vi "Get_Coordinate System.vi"(8 "error in (no error)":errorcluster, 11 "SoftmotionAxis in":refnum<class "SoftmotionAxis.lvclass">) -> (0 "error out":errorcluster, 2 "Coordinate System":refnum<k21>, 3 "SoftmotionAxis out":refnum<class "SoftmotionAxis.lvclass">)   [LabVIEW 2017, in "SoftmotionAxis.lvclass"]
uses:
  SoftmotionAxis.lvclass
  SoftmotionAxis.lvclass/SoftmotionAxis.ctl
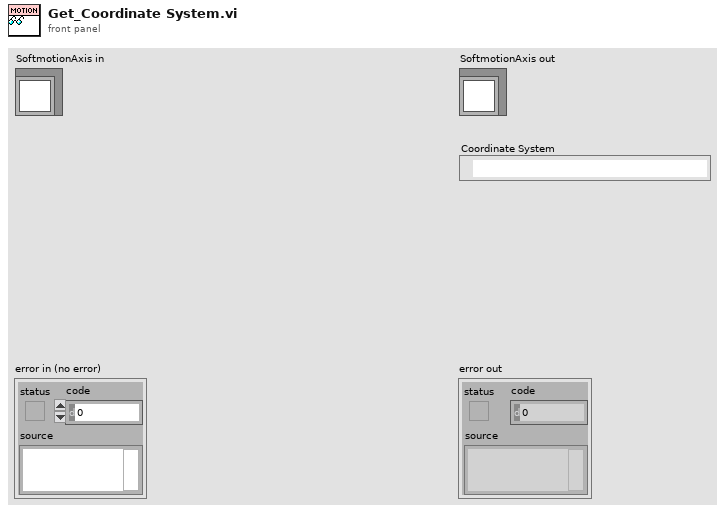
[diagram p1: front panel]
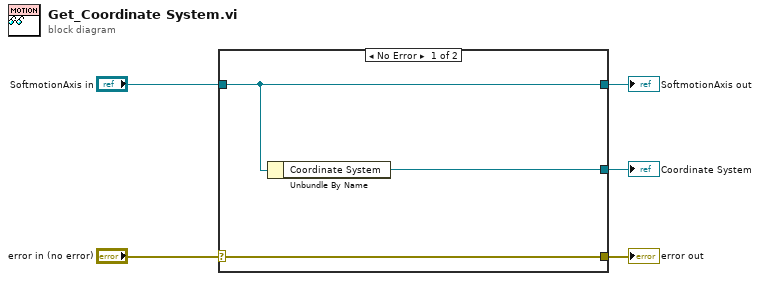
[diagram p0: block diagram]
diagram:
  n1 = case shown="No Error" "error in (no error)" {
    selector: "error in (no error)" -> [w8 w9]
    tunnel: [w8 w9] -> w4
    tunnel: [w7 w10] -> w2
    tunnel: "SoftmotionAxis in" -> [w7 w10]
    tunnel: [w6 _] -> w1
    frame No Error {
      n2 = Unbundle By Name(w7) -> ("Coordinate System"=w6:refnum<k21>)
    }
    frame Error {
    }
  }
  "error out" <- w4
  "SoftmotionAxis out" <- w2
  "Coordinate System" <- w1
